vi "Zero Grabber.vi"() -> (2 "Boolean":bool)   [LabVIEW 2014]
uses:
  Robot Global Data.vi
  <vilib>/Rock Robotics/WPI/SafetyOutput/WPI_SafetyOutputConfigMenu.ctl
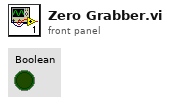
[diagram p1: front panel]
types:
  T1 = typedef "WPI_SafetyOutputConfigMenu.ctl" = enum16{"Enable", "Disable"}
  T2 = typedef "WPI_MotorControlDeviceRef.ctl" = cluster{"DeviceStatus":errorcluster, "Type":T3, "PWM":cluster{"Controller":T4, "PWM Channel":T5, "DeadBand":T6}, "CAN":cluster{"Device Number":u8, "Control Mode":T7, "Semaphore":T8, "Max Vout":dbl, "TalonSRX Control Mode":T9}, "Invert":bool, "TransformRef":T10, "InvTransformRef":T10}
  T3 = typedef "WPI_MotorControlType.ctl" = enum16{"PWM", "CAN", "CANTalonSRX"}
  T4 = typedef "FPGA_TypedefDigitalModule.ctl" = enum16{"Controller 1"}
  T5 = typedef "FPGA_DIOPWMChannel.ctl" = enum8{"PWM 0", "PWM 1", "PWM 2", "PWM 3", "PWM 4", "PWM 5", "PWM 6", "PWM 7", "PWM 8", "PWM 9", "PWM MXP 0", "PWM MXP 1", "PWM MXP 2", "PWM MXP 3", "PWM MXP 4", "PWM MXP 5", "PWM MXP 6", "PWM MXP 7", "PWM MXP 8", "PWM MXP 9", "Invalid"}
  T6 = typedef "WPI_PWMDeadband.ctl" = cluster{"Name":string, "maxPositivePwm":i32, "minPositivePwm":i32, "centerPwm":i32, "maxNegativePwm":i32, "minNegativePwm":i32, "angularRange":u16}
  T7 = typedef "WPI_CANJaguar_ControlMode.ctl" = enum8{"Percent VBus", "Current", "Speed", "Position", "Voltage"}
  T8 = typedef "Semaphore RefNum" = refnum<k1>
  T9 = typedef "WPI_CANTalonSRX_APIControlMode.ctl" = enum8{"Percent VBus", "Speed", "Position", "Slave", "Unchanged / Invalid"}
  T10 = typedef "WPI_PWMTransform_ConPane.ctl" = refnum<vi>
  T11 = typedef "WPI_EncoderDevRef.ctl" = cluster{"DevStatus":errorcluster, "EncoderIndex":T12, "CounterIndex":T13, "DistancePerCount":dbl, "Decoding Type":T14}
  T12 = typedef "FPGA_EncoderIdx.ctl" = enum8{"Enc 0", "Enc 1", "Enc 2", "Enc 3", "Enc 4", "Enc 5", "Enc 6", "Enc 7", "Invalid"}
  T13 = typedef "FPGA_CounterCtrSystemIndex.ctl" = enum8{"Ctr 0", "Ctr 1", "Ctr 2", "Ctr 3", "Ctr 4", "Ctr 5", "Ctr 6", "Ctr 7", "Invalid"}
  T14 = typedef "WPI_EncoderType.ctl" = enum16{"1x", "2x", "4x"}
  T15 = typedef "WPI_DigitalInputDevRef.ctl" = cluster{"DevStatus":errorcluster, "DIO Channel":T16, "Controller":T4}
  T16 = typedef "FPGA_DIOChannel.ctl" = enum8{"DIO 0", "DIO 1", "DIO 2", "DIO 3", "DIO 4", "DIO 5", "DIO 6", "DIO 7", "DIO 8", "DIO 9", "DIO MXP 0", "DIO MXP 1", "DIO MXP 2", "DIO MXP 3", "DIO MXP 4", "DIO MXP 5", "DIO MXP 6", "DIO MXP 7", "DIO MXP 8", "DIO MXP 9", "DIO MXP 10", "DIO MXP 11", "DIO MXP 12", "DIO MXP 13", "DIO MXP 14", "DIO MXP 15", "Invalid"}
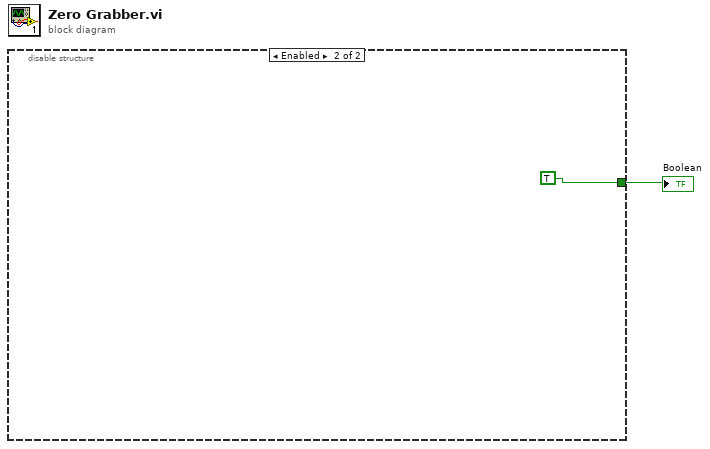
[diagram p0: block diagram]
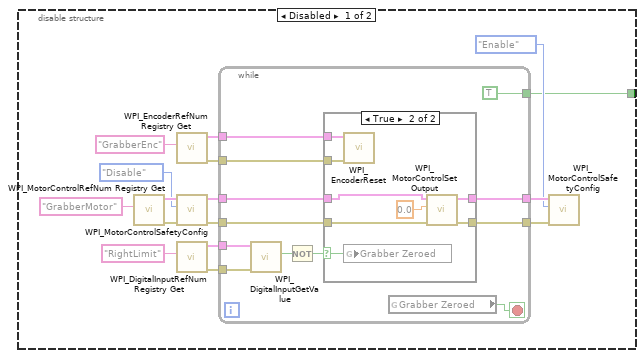
[diagram p2: hidden frame]
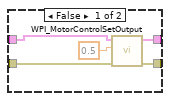
[diagram p3: hidden frame]
diagram:
  n1 = disable-structure shown="Enabled" {
    disable-tunnel: [w2 TRUE] -> w1
    frame Disabled {
      n2 = call <vilib>:"WPI_MotorControlRefNum Registry Get.vi"("refnum name"="GrabberMotor") -> ("error out"=w10:errorcluster, "MotorControlDevRef"=w9:T2)  [unwired: 9 in]
      n3 = call <vilib>:"WPI_EncoderRefNum Registry Get.vi"("refnum name"="GrabberEnc") -> ("error out"=w11:errorcluster, "EncoderDevRef"=w12:T11)  [unwired: 9 in]
      n4 = call <vilib>:"WPI_MotorControlSafetyConfig.vi"("error in (no error)"=w10, "mode"=WPI_SafetyOutputConfigMenu."Disable", "MotorControlDevRef"=w9) -> ("error out"=w7:errorcluster, "MotorControlDevRef"=w8:T2)  [unwired: 7 in]
      n5 = call <vilib>:"WPI_DigitalInputRefNum Registry Get.vi"("refnum name"="RightLimit") -> ("error out"=w14:errorcluster, "DigitalInputDevRef"=w15:T15)  [unwired: 9 in]
      n6 = while {
        tunnel: w15 -> [w26]
        tunnel: w14 -> [w25]
        tunnel: w8 -> [w24]
        tunnel: w7 -> [w23]
        tunnel: [TRUE] -> w2
        tunnel: w12 -> [w21]
        tunnel: w11 -> [w20]
        tunnel: [w19] -> w5
        tunnel: [w18] -> w4
        stop <- w29 stop-if-true
        n7 = call <vilib>:"WPI_DigitalInputGetValue.vi"("error in (no error)"=w25, "DigitalInputDevRef"=w26) -> ("Value"=w28:bool)  [unwired: 7 in, 2 out]
        n8 = Not(x=w28) -> (.not. x?=w27:bool)
        n9 = case shown="True" w27 {
          selector: w27 -> [_ w39]
          tunnel: w24 -> [w33 w41]
          tunnel: w23 -> [w32 w40]
          tunnel: w21 -> [_ w38]
          tunnel: w20 -> [_ w37]
          tunnel: [w31 w36] -> w19
          tunnel: [w30 w35] -> w18
          frame False {
            n10 = call <vilib>:"WPI_MotorControlSetOutput.vi"("error in (no error)"=w32, "Output"=0.5, "MotorControlDevRef"=w33) -> ("error out"=w30:errorcluster, "MotorControlDevRef"=w31:T2)  [unwired: 6 in, 1 out]
          }
          frame True {
            n11 = call <vilib>:"WPI_EncoderReset.vi"("error in (no error)"=w37, "EncoderDevRef"=w38) -> ()  [unwired: 8 in, 2 out]
            n12 = global write "Robot Global Data.vi" "Grabber Zeroed"(w39) -> ()
            n13 = call <vilib>:"WPI_MotorControlSetOutput.vi"("error in (no error)"=w40, "Output"=0.0, "MotorControlDevRef"=w41) -> ("error out"=w35:errorcluster, "MotorControlDevRef"=w36:T2)  [unwired: 6 in, 1 out]
          }
        }
        n14 = global read "Robot Global Data.vi" "Grabber Zeroed"() -> (w29:bool)
      }
      n15 = call <vilib>:"WPI_MotorControlSafetyConfig.vi"("error in (no error)"=w4, "mode"=WPI_SafetyOutputConfigMenu."Enable", "MotorControlDevRef"=w5) -> ()  [unwired: 7 in, 2 out]
    }
    frame Enabled {
    }
  }
  "Boolean" <- w1
